vi "Day 15OLD.vi"() -> ()   [LabVIEW 2021]
uses:
  <vilib>/Utility/file.llb/Read Delimited Spreadsheet (string).vi
panel:
  out "Numeric":i32
  out "min value":i32
  out "Input":i32[][](array[numeric])
  in  "Input File":enum32{"example input", "input"}(radio)
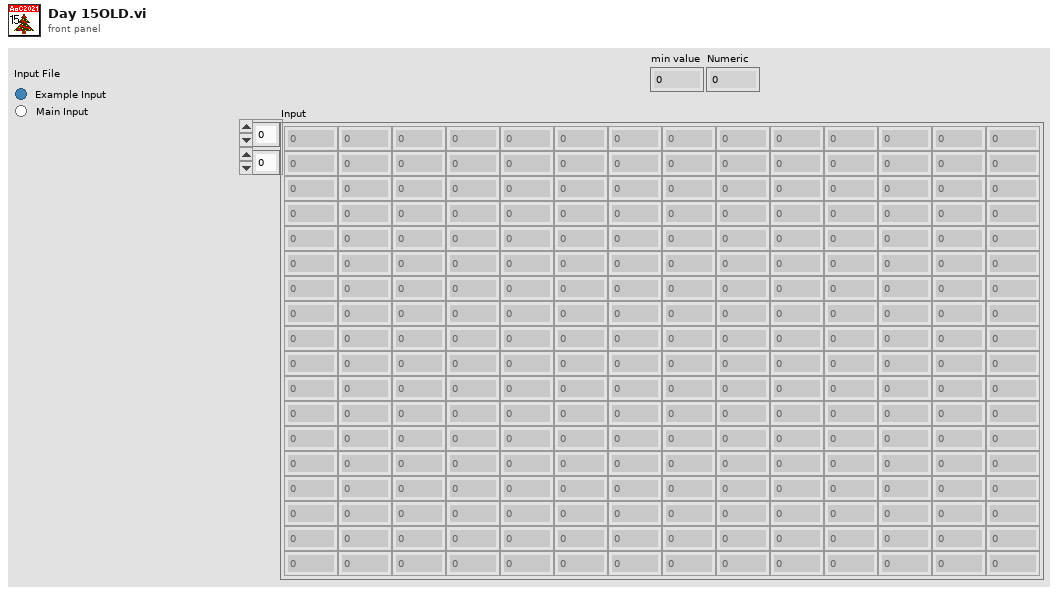
[diagram p1: front panel]
types:
  T1 = typedef "Position.ctl" = cluster{"Row":i32, "Col":i32}
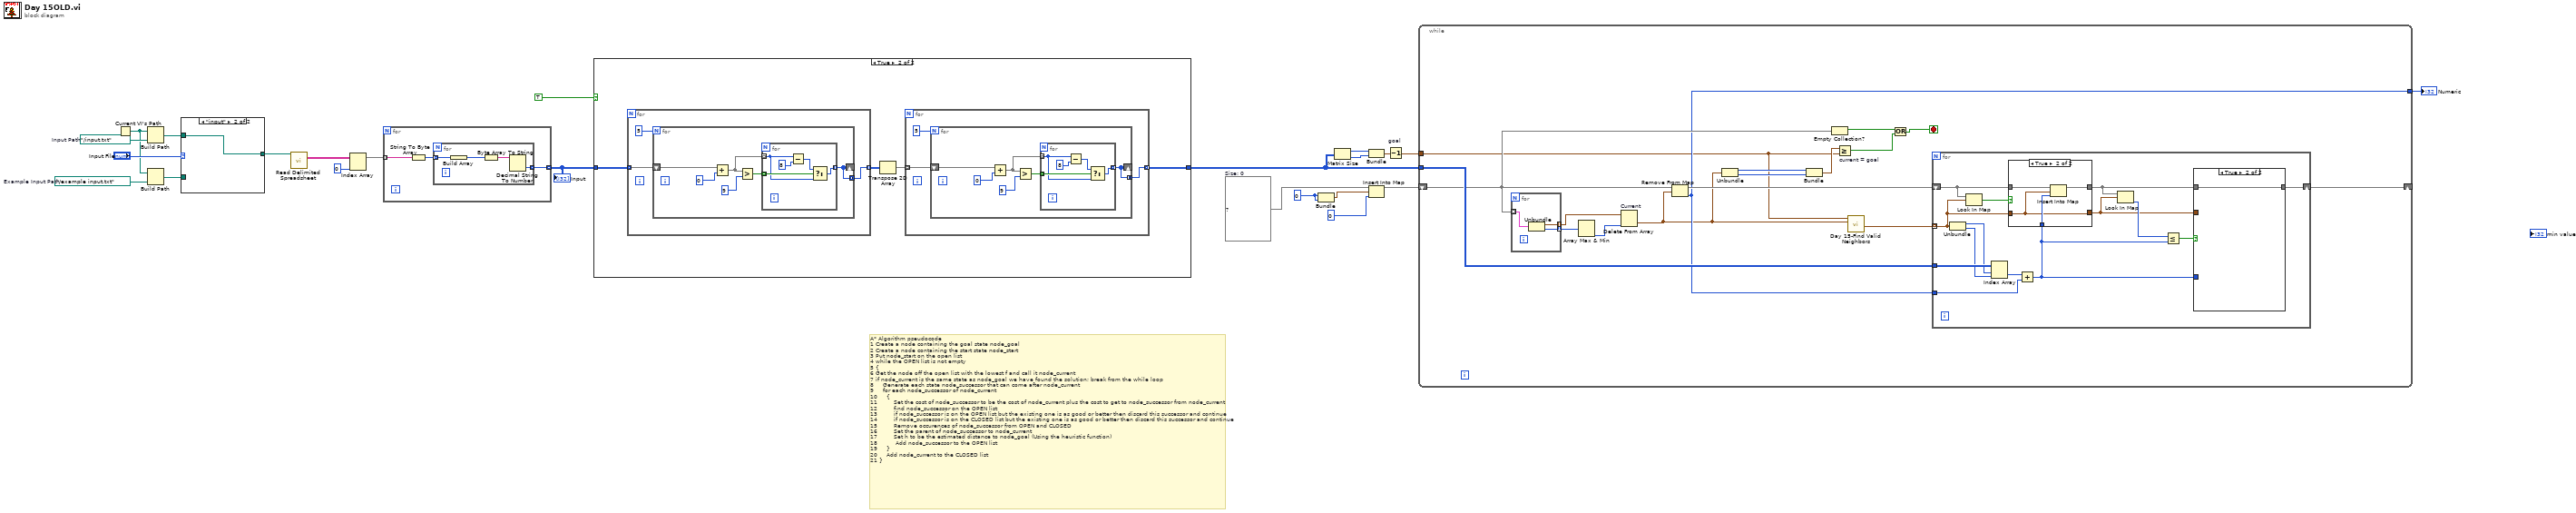
[diagram p0: block diagram]
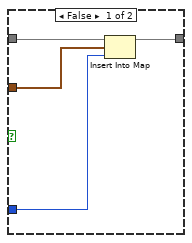
[diagram p4: hidden frame]
diagram:
  w8 = map{cluster{"Row":i32, "Column":i32}, i32} {}  # Size: 0
  w12 = 0 ("index (row)")
  w22 = path "../example input.txt"  # Example Input Path
  w23 = path "../input.txt"  # Input Path
  # "A* Algorithm pseudocode\n1\tCreate a node containing the goal state node_goal\n2\tCreate a node containing the start state node_start\n3\tPut node_start on the open list\n4\twhile the OPEN list is not empty\n5\t{\n6\tGet the node off the open list with the lowest f and call it node_current\n7\tif node_current is the same state as node_goal we have found the solution; break from the while loop\n8\t    Generate each state node_successor that can come after node_current\n9\t    for each node_successor of node_current\n10\t    {\n11\t        Set the cost of node_successor to be the cost of node_current plus the cost to get to node_successor from node_current\n12\t        find node_successor on the OPEN list\n13\t        if node_successor is on the OPEN list but the existing one is as good or better then discard this successor and continue\n14\t        if node_successor is on the CLOSED list but the existing one is as good or better then discard this successor and continue\n15\t        Remove occurences of node_successor from OPEN and CLOSED\n16\t        Set the parent of node_successor to node_current\n17\t        Set h to be the estimated distance to node_goal (Using the heuristic function)\n18\t         Add node_successor to the OPEN list\n19\t    }\n20\t    Add node_current to the CLOSED list\n21\t}"
  n1 = Current VI's Path() -> (path=w17:path)
  n2 = Build Path(base path=w17, name or relative path=w23) -> (appended path=w20:path)
  n3 = Build Path(base path=w17, name or relative path=w22) -> (appended path=w19:path)
  n4 = case shown="\"input\"" "Input File" {
    tunnel: w20 -> [_ w25]
    tunnel: w19 -> [w24 _]
    tunnel: [w24 w25] -> w18
    frame "example input" {
    }
    frame "input" {
    }
  }
  n5 = call-poly <vilib>:"Read Delimited Spreadsheet.vi"("file path (dialog if empty)"=w18) -> ("all rows"=w16:string[][])  [unwired: 9 in, 5 out]
  n6 = Index Array(array=w16, index (col)=0 ("disabled index (col)")) -> (element=w15:string[])  [unwired: 1 in]
  n7 = for {
    tunnel: w15 -> [w28] mode=indexing
    tunnel: [w26] -> w2 mode=indexing
    n8 = String To Byte Array(string=w28) -> (unsigned byte array=w27:u8[])
    n9 = for {
      tunnel: w27 -> [w32] mode=indexing
      tunnel: [w29] -> w26 mode=indexing
      n10 = Build Array(w32) -> (w31:u8[])
      n11 = Byte Array To String(unsigned byte array=w31) -> (string=w30:string)
      n12 = Decimal String To Number(string=w30) -> (number=w29:i32)  [unwired: 2 in, 1 out]
    }
  }
  "Input" <- w2
  n13 = case shown="True" TRUE {
    tunnel: w2 -> [w33 w37]
    tunnel: [w33 w34] -> w1
    frame False {
    }
    frame True {
      n14 = for {
        tunnel: w37 -> [w52] mode=indexing
        tunnel: [w54] -> w36 mode=indexing
        n15 = for {
          N: 5 -> [_]
          tunnel: [w57] -> w54 mode=concatenating
          shift-right: [w57] -> _
          shift-left: w52 -> [w56]
          n16 = Add(x=w56, y=0) -> (x+y=w58:i32[])
          n17 = Greater?(x=w58, y=9) -> (0:w59:bool[])
          n18 = for {
            tunnel: w59 -> [w65] mode=indexing
            tunnel: w58 -> [w64] mode=indexing
            tunnel: [w61] -> w57 mode=indexing
            n19 = Subtract(x=w64, y=8) -> (x-y=w62:i32)
            n20 = Select(t=w62, s=w65, f=w64) -> (s? t:f=w61:i32)
          }
        }
      }
      n21 = Transpose 2D Array(2D array=w36) -> (transposed array=w35:i32[][])
      n22 = for {
        tunnel: w35 -> [w38] mode=indexing
        tunnel: [w40] -> w34 mode=indexing
        n23 = for {
          N: 5 -> [_]
          tunnel: [w43] -> w40 mode=concatenating
          shift-right: [w43] -> _
          shift-left: w38 -> [w42]
          n24 = Add(x=w42, y=0) -> (x+y=w44:i32[])
          n25 = Greater?(x=w44, y=9) -> (0:w45:bool[])
          n26 = for {
            tunnel: w45 -> [w51] mode=indexing
            tunnel: w44 -> [w50] mode=indexing
            tunnel: [w47] -> w43 mode=indexing
            n27 = Subtract(x=w50, y=8) -> (x-y=w48:i32)
            n28 = Select(t=w48, s=w51, f=w50) -> (s? t:f=w47:i32)
          }
        }
      }
    }
  }
  n29 = Bundle("index (row)"=w12, "index (row)"=w12) -> (w7:cluster{"index (row)":i32, "index (row)":i32})  [unwired: 1 in]
  n30 = Matrix Size(0:w1) -> (1:w11:i32, 2:w10:i32)
  n31 = Bundle("number of columns"=w11, "matrix"=w10) -> (w9:cluster{"number of columns":i32, "matrix":i32})  [unwired: 1 in]
  n32 = Insert Into Map(map in=w8, key=w7, value=0 ("index (row)")) -> (map out=w6:map{cluster{"Row":i32, "Column":i32}, i32})  [unwired: 2 out]
  n33 = Decrement "goal"(x=w9) -> (x-1=w13:cluster{"number of columns":i32, "matrix":i32})
  n34 = while {
    tunnel: w1 -> [w76]
    tunnel: w13 -> [w68]
    shift-right: [w70] -> _
    shift-left: w6 -> [w72]
    tunnel: [w69] -> w5
    stop <- w80 stop-if-true
    n35 = for {
      tunnel: w72 -> [w110] mode=indexing
      tunnel: [w109] -> w82 mode=indexing
      tunnel: [w108] -> w74 mode=indexing
      n36 = Unbundle(w110) -> (w108:cluster{"Row":i32, "Column":i32}, w109:i32)
    }
    n37 = Array Max & Min(array=w82) -> (min index (indices)=w78:i32)  [unwired: 3 out]
    n38 = Delete From Array "Current"(array=w74, index=w78) -> (deleted portion=w67:cluster{"Row":i32, "Column":i32})  [unwired: 1 in, 1 out]
    n39 = Remove From Map(10:w67, 11:w72) -> (1:w69:i32, 3:w71:map{cluster{"Row":i32, "Column":i32}, i32})  [unwired: 1 out]
    n40 = Unbundle(w67) -> ("Row"=w77:i32, "Column"=w75:i32)
    n41 = Bundle("Row"=w77, "Column"=w75) -> (w81:cluster{"Row":i32, "Column":i32})  [unwired: 1 in]
    n42 = Empty Collection?(1:w72) -> (0:w73:bool)
    n43 = Greater Or Equal? "current = goal"(x=w81, y=w68) -> (x >= y?=w79:bool)
    n44 = call "Day 15-Find Valid Neighbors.vi"("Current in"=w67, "Goal in"=w68) -> ("All Neighbors"=w66:T1[])  [unwired: 7 in, 2 out]
    n45 = Or(x=w73, y=w79) -> (x .or. y?=w80:bool)
    n46 = for {
      tunnel: w66 -> [w87] mode=indexing
      tunnel: w76 -> [w96]
      tunnel: w69 -> [w95]
      shift-right: [w90] -> w70
      shift-left: w71 -> [w89]
      n47 = Unbundle(w87) -> ("Row"=w93:i32, "Col"=w92:i32)
      n48 = Look In Map(map=w89, key=w87) -> (key not found?=w88:bool)  [unwired: 1 in, 1 out]
      n49 = Index Array(array=w96, index (row)=w93, index (col)=w92) -> (element=w94:i32)
      n50 = Add(x=w94, y=w95) -> (x+y=w86:i32)
      n51 = case shown="True" w88 {
        tunnel: w89 -> [w98 w102]
        tunnel: [w98 w101] -> w85
        tunnel: w87 -> [w97 w99]
        tunnel: w86 -> [_ w100]
        tunnel: [w97 w99] -> w83
        frame False {
        }
        frame True {
          n52 = Insert Into Map(map in=w102, key=w99, value=w100) -> (map out=w101:map{cluster{"Row":i32, "Column":i32}, i32})  [unwired: 2 out]
        }
      }
      n53 = Look In Map(map=w85, key=w83) -> (value=w84:i32)  [unwired: 1 in, 1 out]
      n54 = Less Or Equal?(x=w84, y=w86) -> (x <= y?=w91:bool)
      n55 = case shown="True" w91 {
        tunnel: w85 -> [w106 w107]
        tunnel: [w105 w107] -> w90
        tunnel: w83 -> [w104 _]
        tunnel: w86 -> [w103 _]
        frame False {
          n56 = Insert Into Map(map in=w106, key=w104, value=w103) -> (map out=w105:map{cluster{"Row":i32, "Column":i32}, i32})  [unwired: 2 out]
        }
        frame True {
        }
      }
    }
  }
  "Numeric" <- w5
